vi "Edit.vi"(8 "error in (no error)":errorcluster, 10 "Edit":T1 caption="Edit dialog", 11 "Action in":refnum<class "Move-Timer.lvclass">) -> (0 "error out":errorcluster, 3 "Action out":refnum<class "Move-Timer.lvclass">)   [LabVIEW 2013, in "PowderDeposition.lvlib" / "Move-Timer.lvclass"]
uses:
  Move-Timer.lvclass
  Move-Timer-settings.ctl
  Move-Timer.lvclass/Move-Timer.ctl
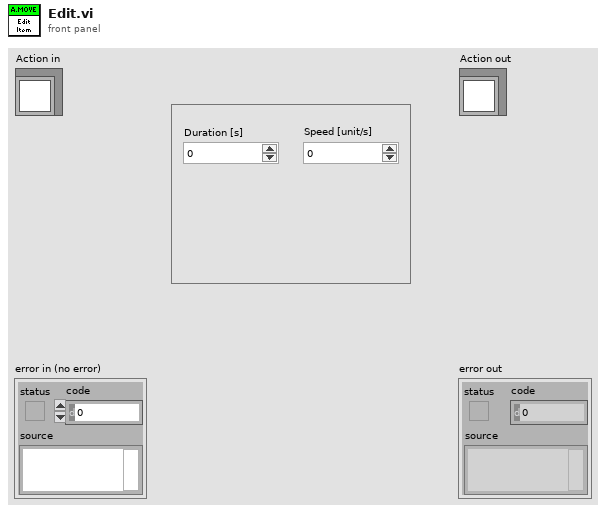
[diagram p1: front panel]
types:
  T1 = typedef "PowderDeposition.lvlib/Move-Timer.lvclass/Move-Timer-settings.ctl" = cluster{"Duration [s]":dbl, "Speed":dbl}
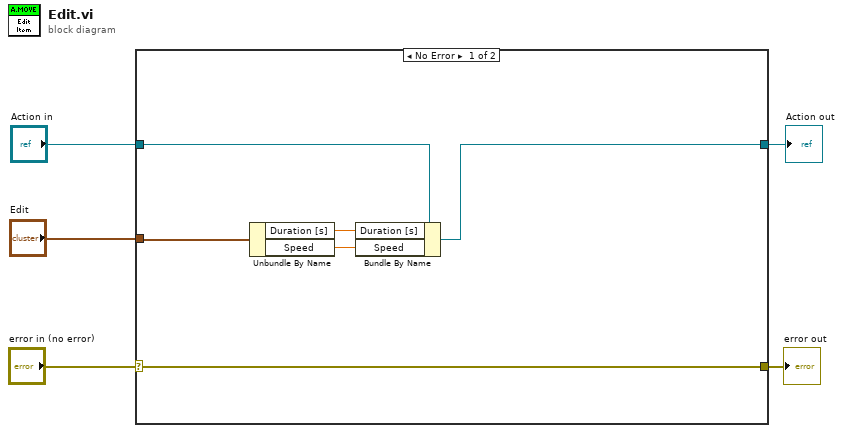
[diagram p0: block diagram]
diagram:
  n1 = case shown="No Error" "error in (no error)" {
    selector: "error in (no error)" -> [w6 w13]
    tunnel: [w6 w13] -> w4
    tunnel: [w7 w12] -> w2
    tunnel: "Action in" -> [w8 w12]
    tunnel: "Edit" -> [w9 _]
    frame No Error {
      n2 = Unbundle By Name(w9) -> ("Duration [s]"=w11:dbl, "Speed"=w10:dbl)
      n3 = Bundle By Name(cluster=w8, "Duration [s]"=w11, "Speed"=w10) -> (w7:refnum<class "Move-Timer.lvclass">)
    }
    frame Error {
    }
  }
  "error out" <- w4
  "Action out" <- w2
